vi "create_images_iteration_directory.vi"(8 "error in (no error)":errorcluster, 10 "Current Iteration":u32, 11 "ExperimentVariables in":refnum<class "ExperimentVariables.lvclass">) -> (0 "error out":errorcluster, 3 "ExperimentVariables out":refnum<class "ExperimentVariables.lvclass">)   [LabVIEW 2012, in "ExperimentVariables.lvclass"]
uses:
  ExperimentVariables.lvclass
  ExperimentVariables.lvclass/ExperimentVariables.ctl
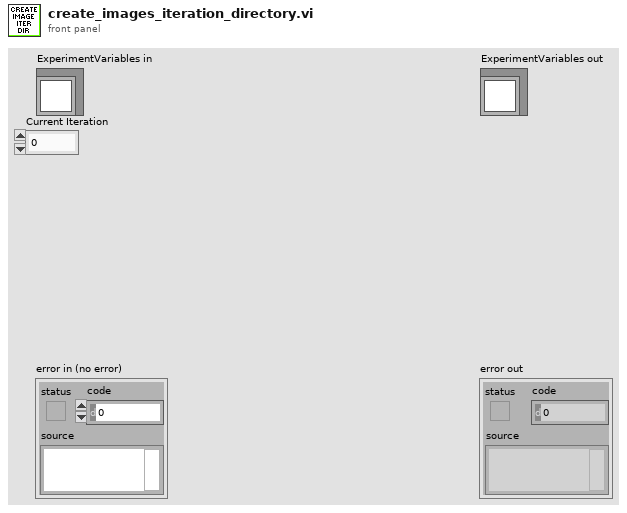
[diagram p1: front panel]
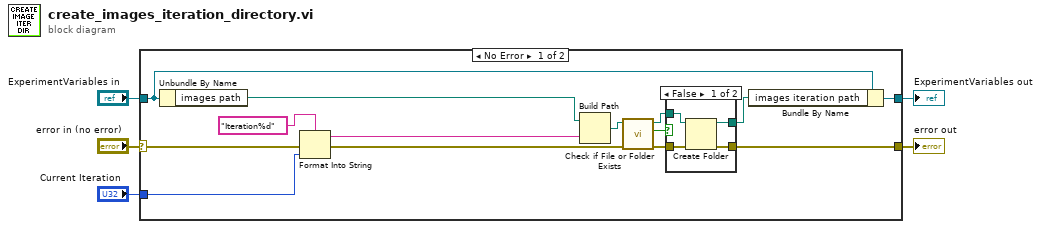
[diagram p0: block diagram]
diagram:
  n1 = case shown="No Error" "error in (no error)" {
    selector: "error in (no error)" -> [w15 w27]
    tunnel: [w9 w27] -> w4
    tunnel: [w6 w26] -> w2
    tunnel: "ExperimentVariables in" -> [w8 w26]
    tunnel: "Current Iteration" -> [w17 _]
    frame No Error {
      n2 = Unbundle By Name(w8) -> ("images path"=w19:path)
      n3 = Format Into String(format string="Iteration%d", error in=w15, w17) -> (resulting string=w16:string, error out=w13:errorcluster)  [unwired: 1 in]
      n4 = Build Path(base path=w19, name or relative path=w16) -> (appended path=w14:path)
      n5 = call <vilib>:"Check if File or Folder Exists.vi"("error in (no error)"=w13, "path"=w14) -> ("error out"=w11:errorcluster, "file or folder exists?"=w12:bool, "dup path"=w10:path)  [unwired: 7 in]
      n6 = case shown="False" w12 {
        tunnel: w11 -> [w23 w24]
        tunnel: w10 -> [w22 w25]
        tunnel: [w21 w25] -> w7
        tunnel: [w20 w24] -> w9
        frame False {
          n7 = Create Folder(path (use dialog)=w22, error in=w23) -> (created path=w21:path, error out=w20:errorcluster)  [unwired: 1 in, 1 out]
        }
        frame True {
        }
      }
      n8 = Bundle By Name(cluster=w8, "images iteration path"=w7) -> (w6:refnum<class "ExperimentVariables.lvclass">)
    }
    frame Error {
    }
  }
  "error out" <- w4
  "ExperimentVariables out" <- w2
